vi "Write.vi"(0 "VISA resource name":refnum<visa-resource-name>, 1 "unsigned byte array":u8[](array[numeric]), 3 "error in (no error)":errorcluster) -> (5 "VISA resource name out":refnum<visa-resource-name>, 8 "error out":errorcluster)   [LabVIEW 2018]
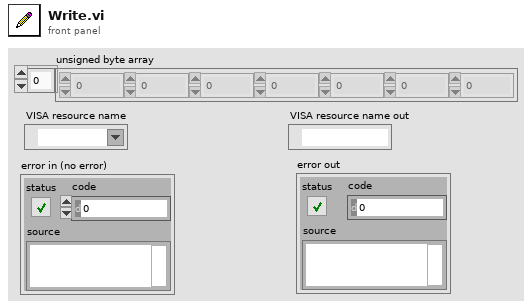
[diagram p1: front panel]
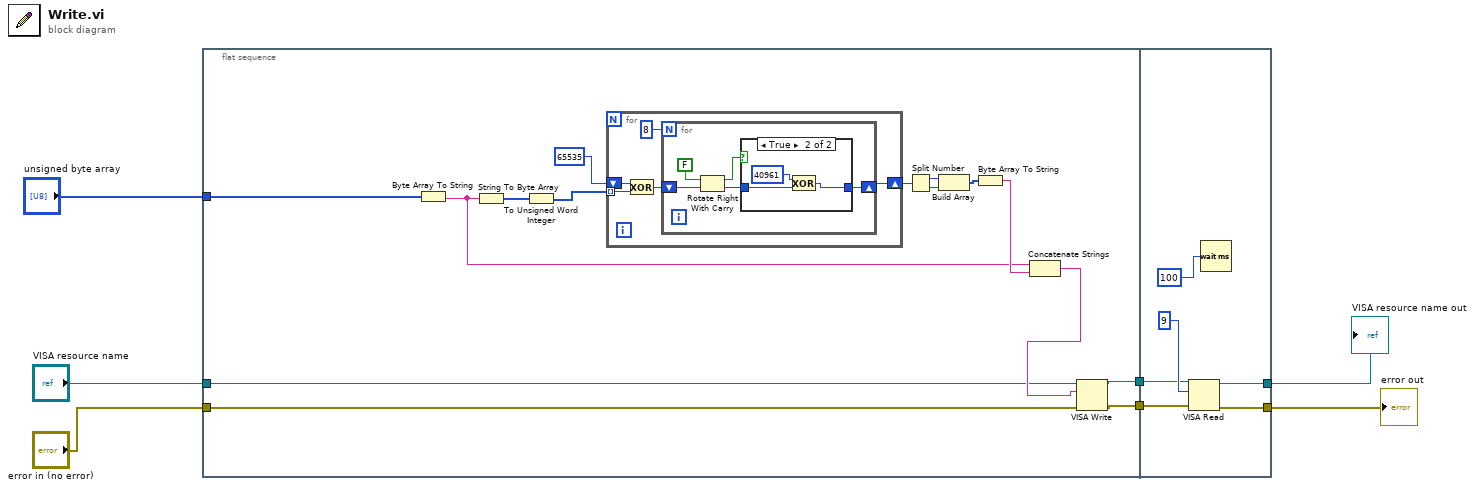
[diagram p0: block diagram]
diagram:
  n1 = flat-sequence {
    tunnel: [w12] -> w7
    tunnel: [w11] -> w6
    tunnel: "unsigned byte array" -> [w10]
    tunnel: "VISA resource name" -> [w9]
    tunnel: "error in (no error)" -> [w8]
    tunnel: w7 -> [w40]
    tunnel: w6 -> [w39]
    tunnel: [w38] -> w3
    tunnel: [w37] -> w4
    frame #0 {
      n2 = Byte Array To String(unsigned byte array=w10) -> (string=w16:string)
      n3 = String To Byte Array(string=w16) -> (unsigned byte array=w20:u8[])
      n4 = To Unsigned Word Integer(number=w20) -> (unsigned 16bit integer=w21:u16[])
      n5 = for {
        shift-right: [w24] -> w22
        shift-left: u16 65535 -> [w25]
        tunnel: w21 -> [w23] mode=indexing
        n6 = Exclusive Or(1:w23, 2:w25) -> (0:w26:u16)
        n7 = for {
          N: 8 -> [_]
          shift-right: [w31] -> w24
          shift-left: w26 -> [w30]
          n8 = Rotate Right With Carry(2:w30, 3:FALSE ("Übertrag")) -> (0:w32:u16, 1:w29:bool)
          n9 = case shown="True" w29 {
            tunnel: w32 -> [w33 w35]
            tunnel: [w33 w34] -> w31
            frame False {
            }
            frame True {
              n10 = Exclusive Or(1:w35, 2:u16 40961) -> (0:w34:u16)
            }
          }
        }
      }
      n11 = Split Number(x=w22) -> (hi(x)=w19:u8, lo(x)=w18:u8)
      n12 = Build Array(w19, w18) -> (w15:u8[])
      n13 = Byte Array To String(unsigned byte array=w15) -> (string=w17:string)
      n14 = Concatenate Strings(w16, w17) -> (w13:string)
      n15 = VISA Write(VISA resource name=w9, write buffer=w13, error in (no error)=w8) -> (VISA resource name out=w12:refnum<visa-resource-name>, error out=w11:errorcluster)  [unwired: 1 out]
    }
    frame #1 {
      n16 = VISA Read(VISA resource name=w40, byte count=u32 9, error in (no error)=w39) -> (VISA resource name out=w38:refnum<visa-resource-name>, error out=w37:errorcluster)  [unwired: 2 out]
      n17 = Wait (ms)(milliseconds to wait=u32 100) -> ()  [unwired: 1 out]
    }
  }
  "error out" <- w4
  "VISA resource name out" <- w3
